vi "oa_Auto Detect RPM Step.vi"(0 "reset?":bool, 5 "speed(RPM)":dbl[](array[numeric]), 7 "start input":dbl, 9 "end input":dbl, 11 "step input":dbl) -> (4 "start output":dbl, 6 "end output":dbl, 8 "step output":dbl, 15 "step found?":bool)   [LabVIEW 2017]
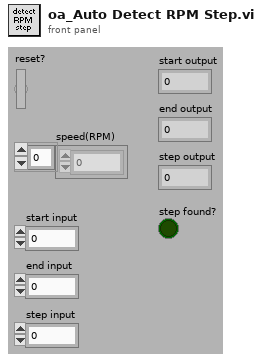
[diagram p1: front panel]
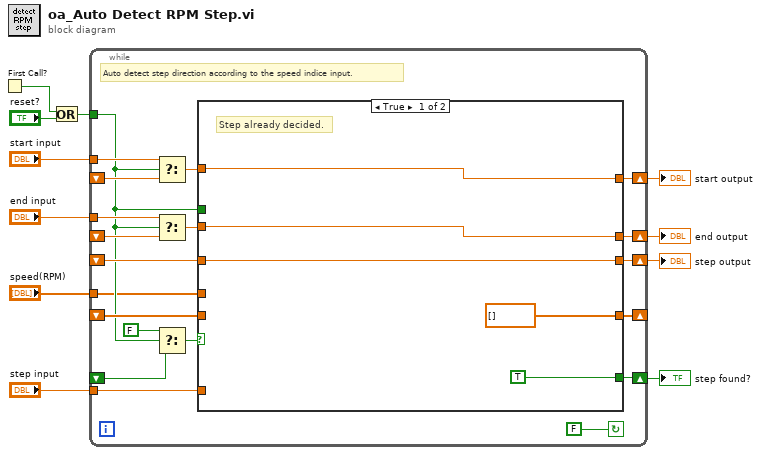
[diagram p0: block diagram]
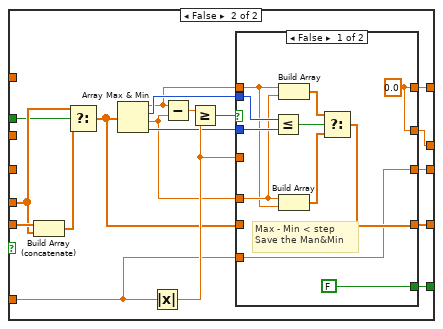
[diagram p2: hidden frame]
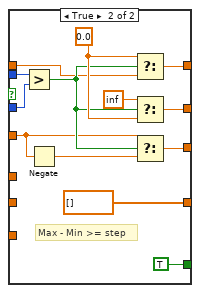
[diagram p3: hidden frame]
diagram:
  n1 = First Call?() -> (First Call?: T/F=w6:bool)
  n2 = Or(x=w6, y="reset?") -> (x .or. y?=w11:bool)
  n3 = while {
    tunnel: w11 -> [w13]
    tunnel: "speed(RPM)" -> [w12]
    shift-right: [w25] -> _
    shift-left: _ -> [w30]
    shift-right: [w24] -> w1
    shift-left: _ -> [w29]
    tunnel: "step input" -> [w27]
    shift-right: [w21] -> w2
    shift-left: _ -> [w20]
    shift-right: [w22] -> w3
    shift-left: _ -> [w16]
    shift-right: [w23] -> w4
    shift-left: _ -> [w19]
    tunnel: "start input" -> [w18]
    tunnel: "end input" -> [w15]
    stop <- FALSE continue-if-true
    # "Auto detect step direction according to the speed indice input."
    n4 = Select(t=w18, s=w13, f=w19) -> (s? t:f=w17:dbl)
    n5 = Select(t=w15, s=w13, f=w16) -> (s? t:f=w14:dbl)
    n6 = Select(t=FALSE, s=w13, f=w29) -> (s? t:f=w26:bool)
    n7 = case shown="True" w26 {
      tunnel: w30 -> [_ w54]
      tunnel: w12 -> [_ w53]
      tunnel: w13 -> [_ w47]
      tunnel: w27 -> [_ w37]
      tunnel: [dbl[] [] ("appended array") w46] -> w25
      tunnel: [TRUE w45] -> w24
      tunnel: [w34 w44] -> w23
      tunnel: [w33 w43] -> w22
      tunnel: [w32 w42] -> w21
      tunnel: w17 -> [w34 _]
      tunnel: w14 -> [w33 _]
      tunnel: w20 -> [w32 _]
      frame True {
        # "Step already decided."
      }
      frame False {
        n8 = Build Array (concatenate)(w54, w53) -> (w48:dbl[])
        n9 = Select(t=w53, s=w47, f=w48) -> (s? t:f=w41:dbl[])
        n10 = Array Max & Min(array=w41) -> (max value=w38:dbl, max index (indices)=w39:i32, min value=w40:dbl, min index (indices)=w51:i32)
        n11 = Absolute Value(x=w37) -> (abs(x)=w52:dbl)
        n12 = Subtract(x=w38, y=w40) -> (x-y=w49:dbl)
        n13 = Greater Or Equal?(x=w49, y=w52) -> (x >= y?=w50:bool)
        n14 = case shown="False" w50 {
          tunnel: [w55 w76] -> w44
          tunnel: [w55 w75] -> w43
          tunnel: [w56 w72] -> w42
          tunnel: w39 -> [w64 w78]
          tunnel: w51 -> [w63 w77]
          tunnel: w52 -> [_ w70]
          tunnel: [w57 dbl[] [] ("appended array")] -> w46
          tunnel: [FALSE TRUE] -> w45
          tunnel: w41 -> [_ _]
          tunnel: w40 -> [w62 _]
          tunnel: w38 -> [w61 w66]
          tunnel: w37 -> [w56 _]
          frame False {
            w55 = 0.0 ("t")
            # "Max - Min < step\nSave the Man&Min"
            n15 = Less Or Equal?(x=w64, y=w63) -> (x <= y?=w60:bool)
            n16 = Build Array(w61, w62) -> (w59:dbl[])
            n17 = Build Array(w62, w61) -> (w58:dbl[])
            n18 = Select(t=w59, s=w60, f=w58) -> (s? t:f=w57:dbl[])
          }
          frame True {
            w73 = 0.0 ("t")
            # "Max - Min >= step"
            n19 = Greater?(x=w78, y=w77) -> (0:w71:bool)
            n20 = Negate(x=w70) -> (-x=w69:dbl)
            n21 = Select(t=w73, s=w71, f=w66) -> (s? t:f=w76:dbl)
            n22 = Select(t=inf ("f"), s=w71, f=w73) -> (s? t:f=w75:dbl)
            n23 = Select(t=w70, s=w71, f=w69) -> (s? t:f=w72:dbl)
          }
        }
      }
    }
  }
  "start output" <- w4
  "end output" <- w3
  "step output" <- w2
  "step found?" <- w1
